vi "dg535 trigger.vi"(1 "external trigger level":sgl min=-2.56 max=2.56 format="%.2f", 2 "burst count":i32=2 min=2 max=32766, 3 "trigger slope":bool, 4 "burst period":i32=4 min=4 max=32766, 5 "input impedance":bool, 6 "error in":errorcluster, 7 "internal/burst trigger rate":dbl=0.001 min=0.001 max=1000000.0 format="%.3f", 8 "trigger":u32(slide) scale=0.0..4.0, 9 "GPIB address":string="15") -> (0 "error out":errorcluster)   [LabVIEW 2013]
doc: "This subVI implements all the trigger commands of the DG535 .\n The trigger mode can be set to internal, external , single shot , burst or line .\n To completely specify the internal mode , the internal trigger rate can be specified . If the DG535 is in the burst mode , the same control is used to specify the burst trigger rate .\n In the external trigger mode , the external trigger level and trigger slope specify the external trigger .\n The burst count specifies the number of pulses which will be in each burst of pulses when in the burst mode and the burst period specifies the number of triggers between the start of each burst of pulses ."
panel:
  # "50 Ohm\nHigh Z"
  # "-ve edge\n+ve  edge"
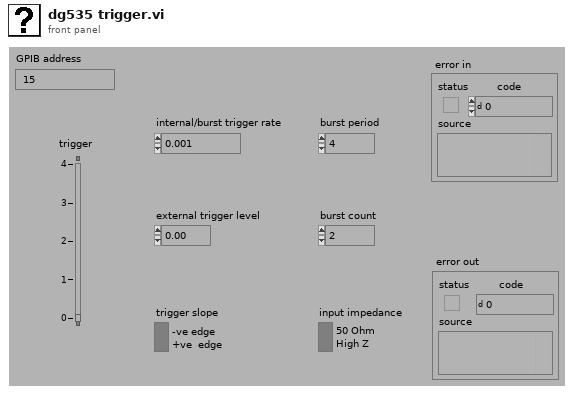
[diagram p1: front panel]
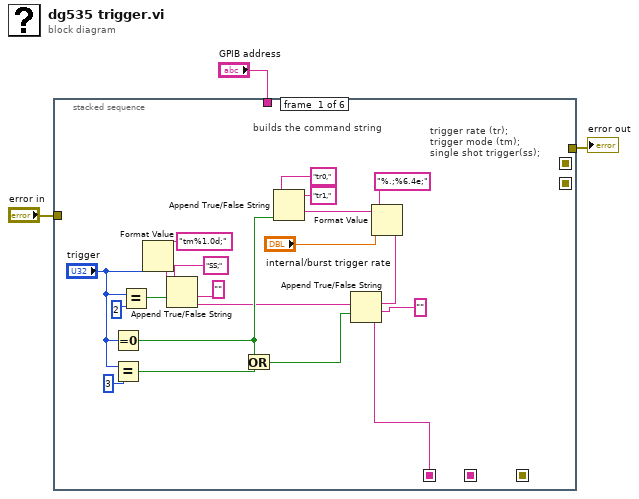
[diagram p0: block diagram]
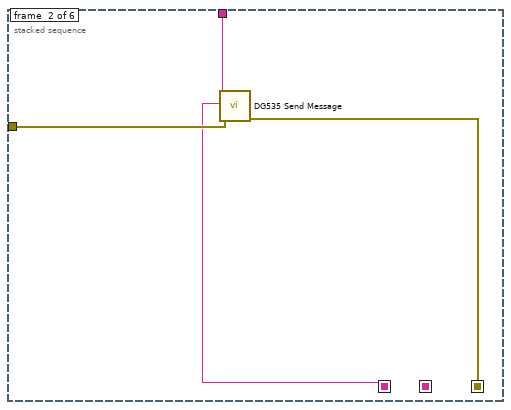
[diagram p2: hidden frame]
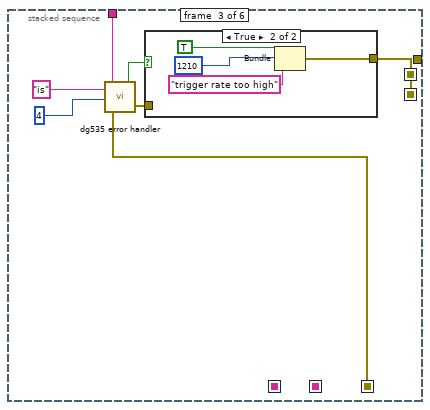
[diagram p3: hidden frame]
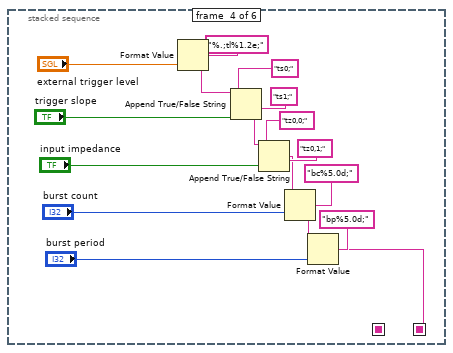
[diagram p5: hidden frame]
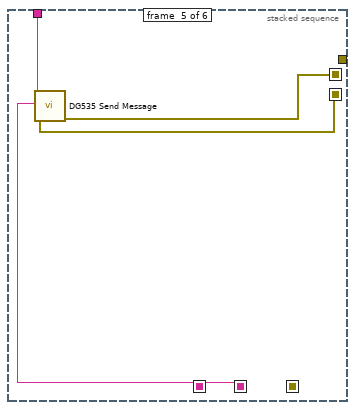
[diagram p6: hidden frame]
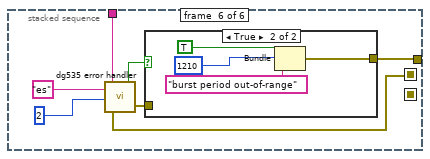
[diagram p7: hidden frame]
diagram:
  n1 = stacked-sequence {
    seq-local: [w4 _ _ _ _ _] -> [_ w24 _ _ _ _]
    seq-local: [_ w25 _ _ _ _] -> [_ _ w28 _ _ _]
    seq-local: [_ _ w29 _ _ _] -> [_ _ _ _ w57 _]
    seq-local: [_ _ _ w40 _ _] -> [_ _ _ _ w58 _]
    seq-local: [_ _ _ _ w59 _] -> [_ _ _ _ _ w61]
    tunnel: "GPIB address" -> [_ w27 w34 _ w60 w67]
    tunnel: "error in" -> [_ w26 _ _ _ _]
    tunnel: [_ _ _ _ _ w62] -> w1
    frame #0 {
      # "trigger rate (tr);\ntrigger mode (tm);\nsingle shot trigger(ss);"
      # "builds the command string"
      n2 = Equal To 0?(x="trigger") -> (x = 0?=w11:bool)
      n3 = Equal?(x="trigger", y=3) -> (x = y?=w15:bool)
      n4 = Equal?(x="trigger", y=2) -> (x = y?=w6:bool)
      n5 = Format Value(format string="tm%1.0d;", value (0)="trigger") -> (output string=w17:string)  [unwired: 1 in]
      n6 = Append True/False String(1:w6, 2:"", 3:"SS;", 4:w17) -> (0:w5:string)
      n7 = Or(x=w11, y=w15) -> (x .or. y?=w14:bool)
      n8 = Append True/False String(1:w11, 2:"tr1,", 3:"tr0,") -> (0:w22:string)  [unwired: 1 in]
      n9 = Format Value(string ("")=w22, format string="%.;%6.4e;", value (0)="internal/burst trigger rate") -> (output string=w12:string)
      n10 = Append True/False String(1:w14, 2:"", 3:w12, 4:w5) -> (0:w4:string)
    }
    frame #1 {
      n11 = call "DG535 Send Message.vi"("address string"=w27, "write buffer"=w24, "error in"=w26) -> ("error out"=w25:errorcluster)  [unwired: 4 in, 2 out]
    }
    frame #2 {
      n12 = call "dg535 error handler.vi"("error in"=w28, "check bit #"=4, "command string"="is", "GPIB address"=w34) -> ("error out"=w30:errorcluster, "error found"=w31:bool)
      n13 = case shown="True" w31 {
        tunnel: [w35 w36] -> w29
        tunnel: w30 -> [w35 _]
        frame False {
        }
        frame True {
          n14 = Bundle(TRUE, 1210, "trigger rate too high") -> (w36:errorcluster)  [unwired: 1 in]
        }
      }
    }
    frame #3 {
      n15 = Format Value(format string="%.;tl%1.2e;", value (0)="external trigger level") -> (output string=w43:string)  [unwired: 1 in]
      n16 = Append True/False String(1:"trigger slope", 2:"ts1;", 3:"ts0;", 4:w43) -> (0:w52:string)
      n17 = Append True/False String(1:"input impedance", 2:"tz0,1;", 3:"tz0,0;", 4:w52) -> (0:w49:string)
      n18 = Format Value(string ("")=w49, format string="bc%5.0d;", value (0)="burst count") -> (output string=w46:string)
      n19 = Format Value(string ("")=w46, format string="bp%5.0d;", value (0)="burst period") -> (output string=w40:string)
    }
    frame #4 {
      n20 = call "DG535 Send Message.vi"("address string"=w60, "write buffer"=w58, "error in"=w57) -> ("error out"=w59:errorcluster)  [unwired: 4 in, 2 out]
    }
    frame #5 {
      n21 = call "dg535 error handler.vi"("error in"=w61, "check bit #"=2, "command string"="es", "GPIB address"=w67) -> ("error out"=w63:errorcluster, "error found"=w64:bool)
      n22 = case shown="True" w64 {
        tunnel: [w68 w69] -> w62
        tunnel: w63 -> [w68 _]
        frame False {
        }
        frame True {
          n23 = Bundle(TRUE, 1210, "burst period out-of-range") -> (w69:errorcluster)  [unwired: 1 in]
        }
      }
    }
  }
  "error out" <- w1
